vi "Calibration Smoothing Tool.vi"(11 "Path In":path) -> (3 "Smoothed?":bool)   [LabVIEW 2020]
uses:
  Type Defs/Cal-Smoothing Data.ctl
  Type Defs/Cal-Smoothing Parameters.ctl
  SubVIs/Calibration Globals.vi
  Instance           1 28Saved   Calibrate Probe Tube .vi
  PXI DAQ VIs/Utility VIs/Array Dimensions (2D).vi
panel:
  out "save signal":bool=TRUE
  out "Dirty?":bool
  out "plot signal":bool=TRUE
  in  "Tab Control":enum32{"Loess", "MA"}(tab)
  in  "MA":cluster{"Iterations":i32, "Length":i32}={"Iterations"=100, "Length"=3} {"Length" min=1 step=1; "Iterations" min=1 step=1}
  in  "Loess":T1={"Length"=21, "Type"=enum."Quadratic", "Robust"=TRUE} {"Length" min=1 step=1}
  in  "Method":enum16{"Moving average", "Loess"}(ring)=enum."Loess"
  in  "Exit Button":bool
  in  "Apply Button":bool
  in  "Save Button":bool
  in  "Clear Button":bool
  in  "Open Button":bool
  out "exit signal":bool=TRUE
  out "Path":path=path "C:/Data/Probe Tube Calibrations/SN31_ProbeTube.calib"
  out "PT phase graph":cluster{"PTC Mag":dbl[], "PTC Phase":dbl[]}[](graph)
  out "Mag Graph":cluster{"Numeric":dbl, dbl, dbl[][]}(graph)
  # "Smoothing parameters"
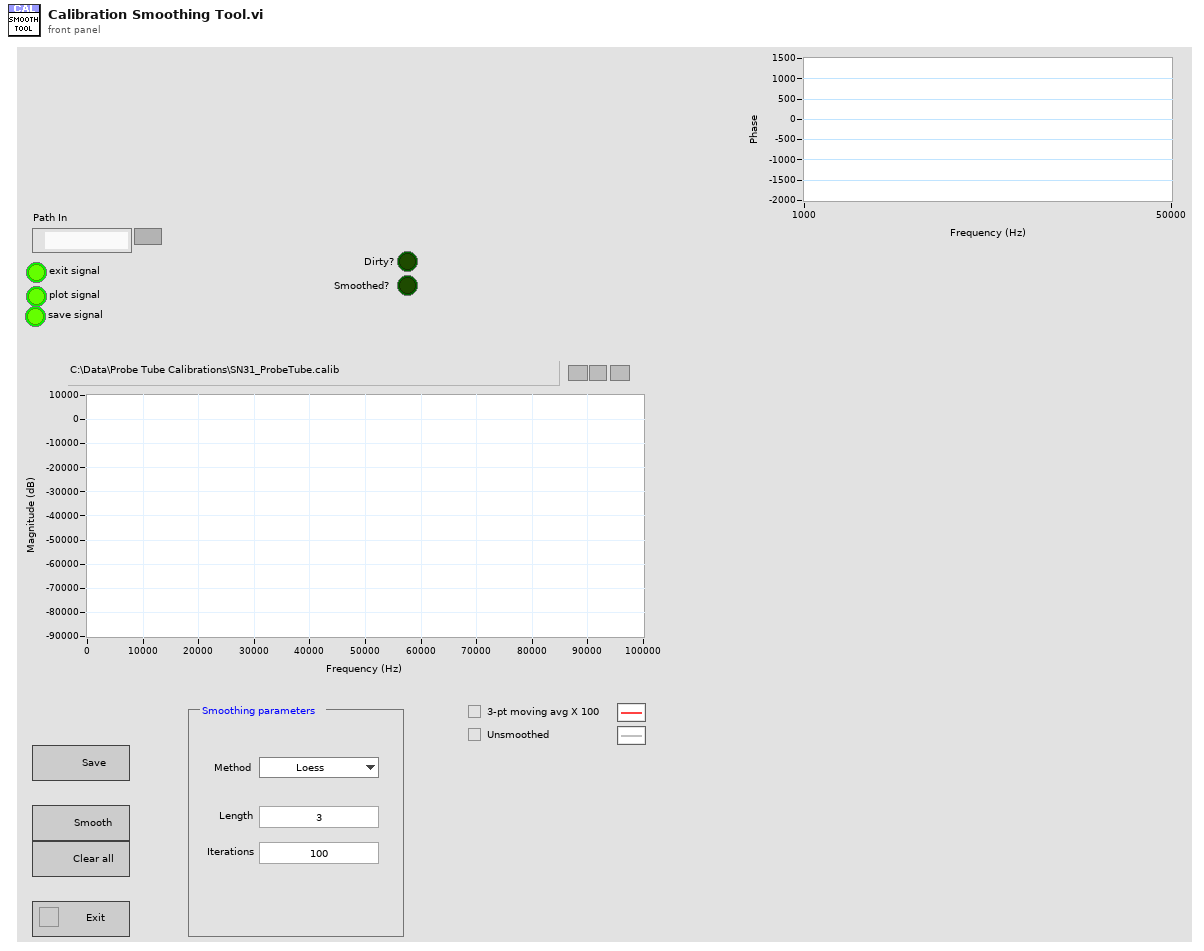
[diagram p1: front panel]
types:
  T1 = cluster{"Length":i32, "Type":enum16{"Linear", "Quadratic"}, "Robust":bool}
  T2 = typedef "Cal-Smoothing Data.ctl" = cluster{"Data":cluster{"x0":dbl, "dx":dbl, "Array":dbl[][]}, "Labels":string[], "Smooth Params":T3}
  T3 = typedef "Cal-Smoothing Parameters.ctl" = cluster{"Method":enum16{"None", "Moving average", "Loess"}, "MA":cluster{"Iterations":i32, "Length":i32}, "Loess":cluster{"Length":i32, "Type":enum16{"Linear", "Quadratic"}, "Robust":bool}}
  T4 = enum16{"Left Button", "Center Button", "Right Button", "Window Close"}
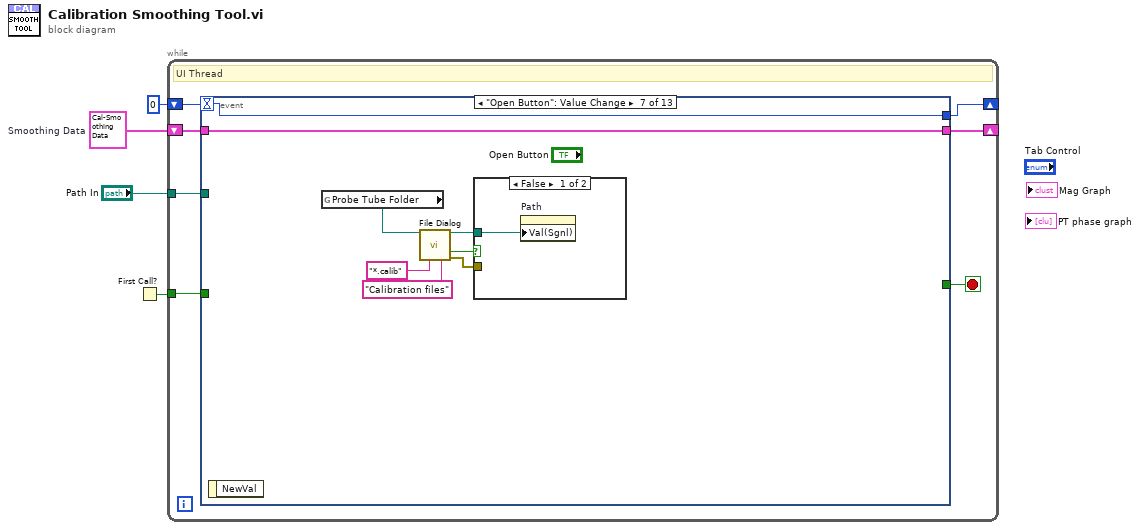
[diagram p0: block diagram]
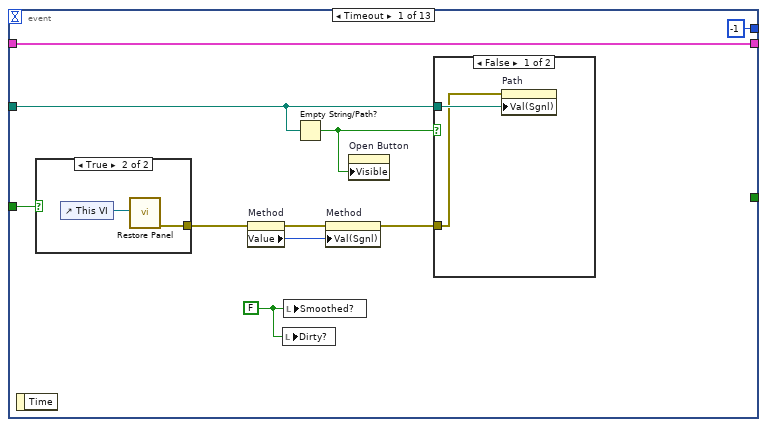
[diagram p2: hidden frame]
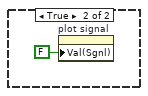
[diagram p3: hidden frame]
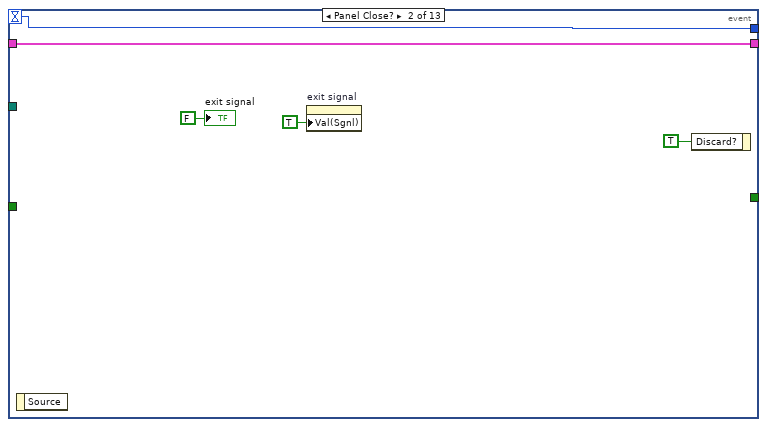
[diagram p5: hidden frame]
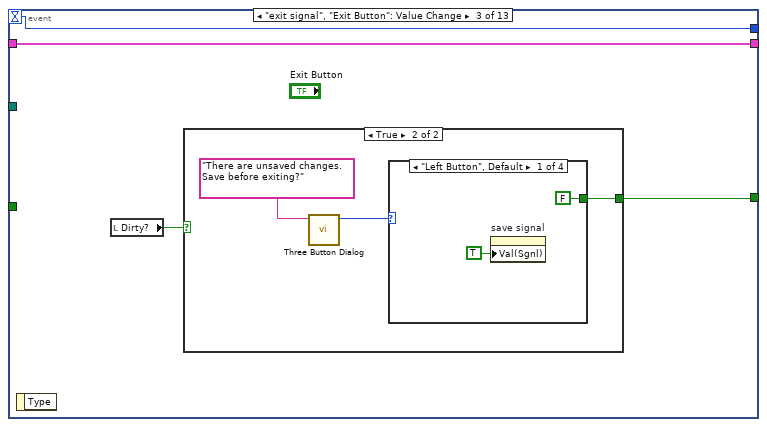
[diagram p6: hidden frame]
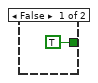
[diagram p7: hidden frame]
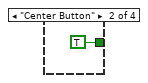
[diagram p8: hidden frame]
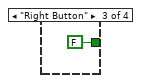
[diagram p9: hidden frame]
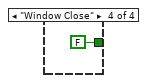
[diagram p10: hidden frame]
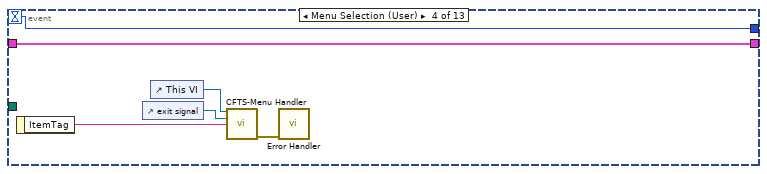
[diagram p11: hidden frame]
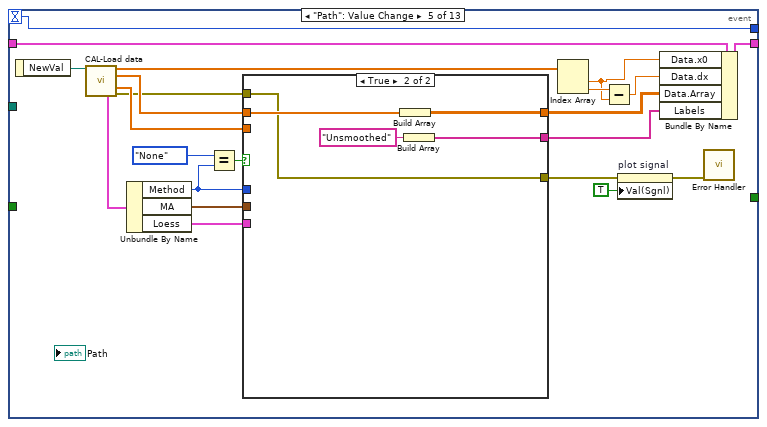
[diagram p12: hidden frame]
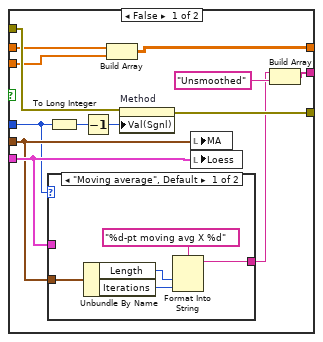
[diagram p13: hidden frame]
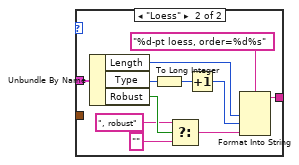
[diagram p14: hidden frame]
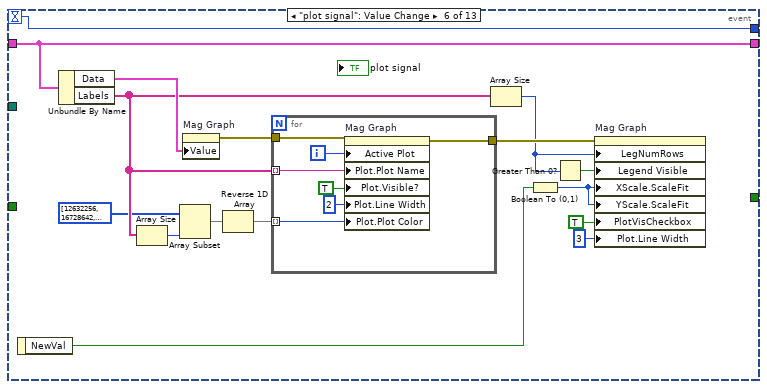
[diagram p15: hidden frame]
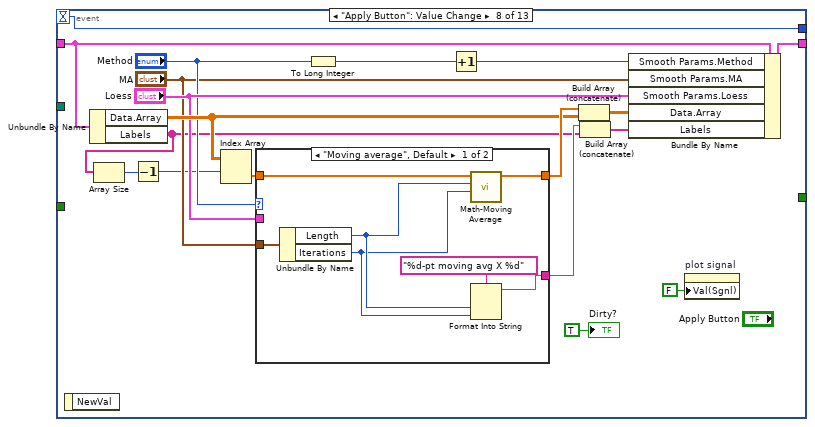
[diagram p17: hidden frame]
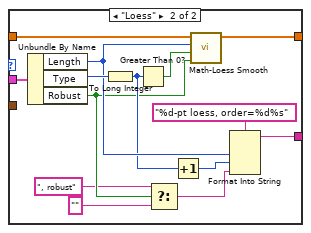
[diagram p18: hidden frame]
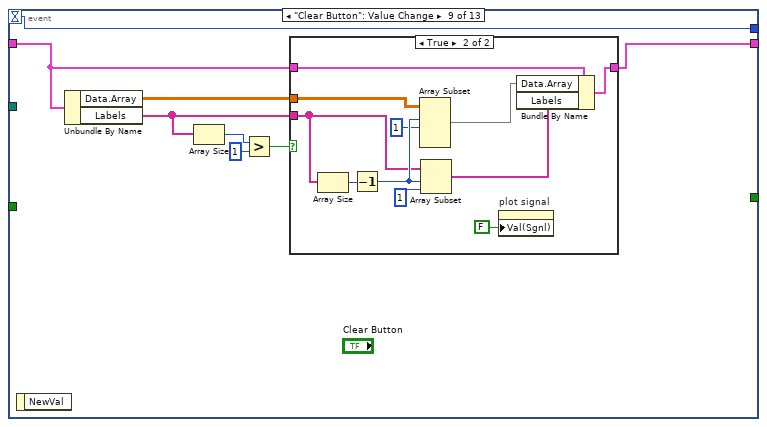
[diagram p19: hidden frame]
diagram:
  w2 = T2 {"Data"={"x0"=0.0, "dx"=0.0, "Array"=[]}, "Labels"=[], "Smooth Params"={"Method"=enum."Loess", "MA"={"Iterations"=100, "Length"=3}, "Loess"={"Length"=21, "Type"=enum."Quadratic", "Robust"=TRUE}}}  # Smoothing Data
  n1 = First Call?() -> (First Call?: T/F=w3:bool)
  n2 = while {
    shift-right: [w9] -> _
    shift-left: 0 -> [w10]
    tunnel: w3 -> [w8]
    shift-right: [w6] -> _
    shift-left: w2 -> [w7]
    tunnel: "Path In" -> [w5]
    stop <- w11 stop-if-true
    # "UI Thread"
    n3 = event shown="[6] \"Open Button\": Value Change" {
      selector: _ -> [_ _ _ _ _ _ _ _ _ _ _ _ _]
      dyn-events: _ -> [_ _ _ _ _ _ _ _ _ _ _ _ _]
      timeout: w10 -> [_ w30 w35 w50 w72 w122 w132 w157 w186 w201 w210 w228 w230]
      tunnel: [_ _ w33 _ _ _ _ _ _ _ w202 _ _] -> w11
      tunnel: [-1 w30 w35 w50 w72 w122 w132 w157 w186 w201 w210 w228 w230] -> w9
      tunnel: w8 -> [w20 _ _ _ _ _ _ _ _ _ _ _ _]
      tunnel: w7 -> [w19 w27 w32 w45 w67 w121 w131 w154 w185 w200 w209 w225 w229]
      tunnel: [w19 w27 w32 w45 w66 w121 w131 w152 w183 w200 w209 w225 w229] -> w6
      tunnel: w5 -> [w15 _ _ _ _ _ _ _ _ _ _ _ _]
      event Timeout {
        w14 = FALSE ("Smoothed?")
        n4 = event-data() -> ()  [unwired: 1 in, 1 out]
        n5 = case shown="True" w20 {
          tunnel: [_ w25] -> w18
          frame False {
          }
          frame True {
            n6 = control-ref of="This VI"() -> (w26:refnum<vi>)
            n7 = call "Restore Panel.vi"("VI reference"=w26) -> ("error out"=w25:errorcluster)  [unwired: 10 in]
          }
        }
        n8 = property on="Method" class="Enum (strict)"(error in=w18) -> (error out=w17:errorcluster, "Value"=w16:enum16{"Moving average", "Loess"})  [unwired: 1 in, 1 out]
        n9 = local write "Dirty?"(w14) -> ()
        n10 = local write "Smoothed?"(w14) -> ()
        n11 = Empty String/Path?(string/path=w15) -> (empty?=w12:bool)
        n12 = property on="Method" class="Enum (strict)"(error in=w17, "Val(Sgnl)"=w16) -> (error out=w13:errorcluster)  [unwired: 1 in, 1 out]
        n13 = property on="Open Button" class="Bool"("Visible"=w12) -> ()  [unwired: 2 in, 2 out]
        n14 = case shown="False" w12 {
          tunnel: w15 -> [w23 _]
          tunnel: w13 -> [w22 _]
          frame False {
            n15 = property on="Path" class="Path"(error in=w22, "Val(Sgnl)"=w23) -> ()  [unwired: 1 in, 2 out]
          }
          frame True {
            n16 = property on="plot signal" class="Bool (strict)"("Val(Sgnl)"=FALSE ("Value (Signaling)")) -> ()  [unwired: 2 in, 2 out]
          }
        }
      }
      event Panel Close? {
        n17 = event-data() -> ()  [unwired: 1 in, 1 out]
        n18 = property on="exit signal" class="Bool (strict)"("Val(Sgnl)"=TRUE ("Value (Signaling)")) -> ()  [unwired: 2 in, 2 out]
        n19 = event-data("Discard?"=TRUE) -> ()  [unwired: 1 in, 1 out]
        "exit signal" <- FALSE ("exit signal")
      }
      event "exit signal", "Exit Button": Value Change {
        n20 = event-data() -> ()  [unwired: 1 in, 1 out]
        n21 = local read "Dirty?"() -> (w34:bool)
        n22 = case shown="True" w34 {
          tunnel: [TRUE w37] -> w33
          frame False {
          }
          frame True {
            n23 = call <vilib>:"Three Button Dialog.vi"("message"="There are unsaved changes. Save before exiting?") -> ("Which Button?"=w38:T4)  [unwired: 10 in]
            n24 = case shown="\"Left Button\", Default" w38 {
              tunnel: [FALSE TRUE FALSE FALSE] -> w37
              frame "Left Button", Default {
                n25 = property on="save signal" class="Bool (strict)"("Val(Sgnl)"=TRUE ("Value (Signaling)")) -> ()  [unwired: 2 in, 2 out]
              }
              frame "Center Button" {
              }
              frame "Right Button" {
              }
              frame "Window Close" {
              }
            }
          }
        }
      }
      event Menu Selection (User) {
        n26 = event-data() -> ("ItemTag"=w47:string)  [unwired: 1 in]
        n27 = control-ref of="exit signal"() -> (w46:refnum<vi>)
        n28 = control-ref of="This VI"() -> (w49:refnum<vi>)
        n29 = call "CFTS-Menu Handler.vi"("VI Refnum"=w49, "Return Refnum"=w46, "ItemTag"=w47) -> ("error out"=w48:errorcluster)  [unwired: 11 in, 1 out]
        n30 = call "Error Handler.vi"("error in (no error)"=w48) -> ()  [unwired: 13 in, 2 out]
      }
      event "Path": Value Change {
        n31 = event-data() -> ("NewVal"=w71:path)  [unwired: 1 in]
        n32 = call "CAL-Load data.vi"("user path"=w71) -> ("Smooth Params"=w59:T3, "Frequency (Hz)"=w69:dbl[], "Mag"=w68:dbl[], "Unsmoothed Mag"=w56:dbl[], "error out"=w52:errorcluster)  [unwired: 7 in, 3 out]
        n33 = Unbundle By Name(w59) -> ("Method"=w53:enum16{"None", "Moving average", "Loess"}, "MA"=w55:cluster{"Iterations":i32, "Length":i32}, "Loess"=w54:T1)
        n34 = Equal?(x=enum16{"None", "Moving average", "Loess"}."None", y=w53) -> (x = y?=w57:bool)
        n35 = case shown="True" w57 {
          tunnel: w68 -> [w84 w106]
          tunnel: [w82 w105] -> w63
          tunnel: [w80 w103] -> w60
          tunnel: w56 -> [w83 _]
          tunnel: w55 -> [w75 _]
          tunnel: w54 -> [w76 _]
          tunnel: w53 -> [w74 _]
          tunnel: w52 -> [w85 w102]
          tunnel: [w77 w102] -> w51
          frame False {
            n36 = case shown="\"Moving average\", Default" w74 {
              tunnel: w76 -> [_ w100]
              tunnel: w75 -> [w90 _]
              tunnel: [w88 w98] -> w73
              frame "Moving average", Default {
                n37 = Unbundle By Name(w90) -> ("Length"=w87:i32, "Iterations"=w86:i32)
                n38 = Format Into String(format string="%d-pt moving avg X %d", w87, w86) -> (resulting string=w88:string)  [unwired: 2 in, 1 out]
              }
              frame "Loess" {
                n39 = Unbundle By Name(w100) -> ("Length"=w97:i32, "Type"=w101:enum16{"Linear", "Quadratic"}, "Robust"=w93:bool)
                n40 = To Long Integer(number=w101) -> (32bit integer=w96:i32)
                n41 = Select(t=", robust", s=w93, f="") -> (s? t:f=w94:string)
                n42 = Increment(x=w96) -> (x+1=w95:i32)
                n43 = Format Into String(format string="%d-pt loess, order=%d%s", w97, w95, w94) -> (resulting string=w98:string)  [unwired: 2 in, 1 out]
              }
            }
            n44 = To Long Integer(number=w74) -> (32bit integer=w79:i32)
            n45 = Decrement(x=w79) -> (x-1=w78:i32)
            n46 = Build Array(w84, w83) -> (w82:dbl[][])
            n47 = property on="Method" class="Enum (strict)"(error in=w85, "Val(Sgnl)"=w78) -> (error out=w77:errorcluster)  [unwired: 1 in, 1 out]
            n48 = local write "MA"(w75) -> ()
            n49 = local write "Loess"(w76) -> ()
            n50 = Build Array(w73, "Unsmoothed") -> (w80:string[])
          }
          frame True {
            n51 = Build Array(w106) -> (w105:dbl[][])
            n52 = Build Array("Unsmoothed" ("String")) -> (w103:string[])
          }
        }
        n53 = Index Array(array=w69) -> (element #1=w65:dbl, element #2=w70:dbl)  [unwired: 2 in]
        n54 = Subtract(x=w70, y=w65) -> (x-y=w64:dbl)
        n55 = property on="plot signal" class="Bool (strict)"(error in=w51, "Val(Sgnl)"=TRUE ("Value (Signaling)")) -> (error out=w62:errorcluster)  [unwired: 1 in, 1 out]
        n56 = Bundle By Name(cluster=w67, "Data.x0"=w65, "Data.dx"=w64, "Data.Array"=w63, "Labels"=w60) -> (w66:T2)
        n57 = call "Error Handler.vi"("error in (no error)"=w62) -> ()  [unwired: 13 in, 2 out]
      }
      event "plot signal": Value Change {
        n58 = event-data() -> ("NewVal"=w119:bool)  [unwired: 1 in]
        n59 = Unbundle By Name(w121) -> ("Data"=w117:cluster{"x0":dbl, "dx":dbl, "Array":dbl[][]}, "Labels"=w111:string[])
        n60 = Array Size(array=w111) -> (size(s)=w110:i32)
        n61 = Array Subset(array=u32[] [12632256, 16728642, 982784, 4375295, 13827953, 13457919, 16757522, 4343295, 16728758, 5898228] ("Array"), length=w110) -> (w108:u32[])  [unwired: 1 in]
        n62 = property on="Mag Graph" class="WFGraph (strict)"("Value"=w117) -> (error out=w118:errorcluster)  [unwired: 2 in, 1 out]
        n63 = Reverse 1D Array(array=w108) -> (reversed array=w107:u32[])
        n64 = for {
          tunnel: w111 -> [w128] mode=indexing
          tunnel: [w127] -> w120
          tunnel: w118 -> [w126]
          tunnel: w107 -> [w123] mode=indexing
          i -> [w129]
          n65 = property on="Mag Graph" class="WFGraph (strict)"(error in=w126, "Active Plot"=w129, "Plot.Plot Name"=w128, "Plot.Visible?"=TRUE ("Plot.Visible"), "Plot.Line Width"=u8 2, "Plot.Plot Color"=w123) -> (error out=w127:errorcluster)  [unwired: 1 in, 1 out]
        }
        n66 = Array Size(array=w111) -> (size(s)=w114:i32)
        n67 = Boolean To (0,1)(Boolean=w119) -> (0, 1=w113:i16)
        n68 = Greater Than 0?(x=w114) -> (x > 0?=w115:bool)
        n69 = property on="Mag Graph" class="WFGraph (strict)"(error in=w120, "LegNumRows"=w114, "Legend Visible"=w115, "XScale.ScaleFit"=w113, "YScale.ScaleFit"=w113, "PlotVisCheckbox"=TRUE ("Legend:Plot Visibility Checkbox Visible"), "Plot.Line Width"=u8 3) -> ()  [unwired: 1 in, 2 out]
      }
      event "Open Button": Value Change {
        n70 = event-data() -> ()  [unwired: 1 in, 1 out]
        n71 = global read "Calibration Globals.vi" "Probe Tube Folder"() -> (w133:path)
        n72 = call "File Dialog"("start path"=w133, "pattern (all files)"="*.calib", "pattern label"="Calibration files") -> ("selected path"=w136:path, "cancelled"=w137:bool, "error out"=w130:errorcluster)  [unwired: 9 in, 1 out]
        n73 = case shown="False" w137 {
          tunnel: w136 -> [w138 _]
          tunnel: w130 -> [_ _]
          frame False {
            n74 = property on="Path" class="Path"("Val(Sgnl)"=w138) -> ()  [unwired: 2 in, 2 out]
          }
          frame True {
          }
        }
      }
      event "Apply Button": Value Change {
        n75 = event-data() -> ()  [unwired: 1 in, 1 out]
        n76 = Unbundle By Name(w154) -> ("Data.Array"=w153:dbl[][], "Labels"=w141:string[])
        n77 = Array Size(array=w141) -> (size(s)=w140:i32)
        n78 = Decrement(x=w140) -> (x-1=w139:i32)
        n79 = Index Array(array=w153, index (row)=w139) -> (element=w156:dbl[])  [unwired: 1 in]
        n80 = case shown="\"Moving average\", Default" "Method" {
          tunnel: w156 -> [w163 w178]
          tunnel: [w162 w177] -> w155
          tunnel: "Loess" -> [_ w174]
          tunnel: "MA" -> [w164 _]
          tunnel: [w160 w172] -> w145
          frame "Moving average", Default {
            n81 = Unbundle By Name(w164) -> ("Length"=w159:i32, "Iterations"=w158:i32)
            n82 = call "Math-Moving Average.vi"("Iterations"=w158, "Length"=w159, "Array in"=w163) -> ("Array out"=w162:dbl[])  [unwired: 8 in]
            n83 = Format Into String(format string="%d-pt moving avg X %d", w159, w158) -> (resulting string=w160:string)  [unwired: 2 in, 1 out]
          }
          frame "Loess" {
            n84 = Unbundle By Name(w174) -> ("Length"=w171:i32, "Type"=w176:enum16{"Linear", "Quadratic"}, "Robust"=w167:bool)
            n85 = To Long Integer(number=w176) -> (32bit integer=w170:i32)
            n86 = Greater Than 0?(x=w170) -> (x > 0?=w175:bool)
            n87 = Select(t=", robust", s=w167, f="") -> (s? t:f=w168:string)
            n88 = Increment(x=w170) -> (x+1=w169:i32)
            n89 = call "Math-Loess Smooth.vi"("Robust?"=w167, "Quadratic?"=w175, "Span"=w171, "Array"=w178) -> ("Smoothed Array"=w177:dbl[])  [unwired: 7 in]
            n90 = Format Into String(format string="%d-pt loess, order=%d%s", w171, w169, w168) -> (resulting string=w172:string)  [unwired: 2 in, 1 out]
          }
        }
        n91 = To Long Integer(number="Method") -> (32bit integer=w144:i32)
        n92 = Increment(x=w144) -> (x+1=w143:i32)
        n93 = Build Array (concatenate)(w155, w153) -> (w149:dbl[][])
        n94 = Build Array (concatenate)(w145, w141) -> (w148:string[])
        n95 = Bundle By Name(cluster=w154, "Smooth Params.Method"=w143, "Smooth Params.MA"="MA", "Smooth Params.Loess"="Loess", "Data.Array"=w149, "Labels"=w148) -> (w152:T2)
        n96 = property on="plot signal" class="Bool (strict)"("Val(Sgnl)"=FALSE ("Value (Signaling)")) -> ()  [unwired: 2 in, 2 out]
        "Dirty?" <- TRUE ("Dirty?")
      }
      event "Clear Button": Value Change {
        n97 = event-data() -> ()  [unwired: 1 in, 1 out]
        n98 = Unbundle By Name(w185) -> ("Data.Array"=w184:dbl[][], "Labels"=w180:string[])
        n99 = Array Size(array=w180) -> (size(s)=w181:i32)
        n100 = Greater?(x=w181, y=1) -> (0:w179:bool)
        n101 = case shown="True" w179 {
          tunnel: w185 -> [w187 w198]
          tunnel: w184 -> [_ w195]
          tunnel: w180 -> [_ w194]
          tunnel: [w187 w191] -> w183
          frame False {
          }
          frame True {
            n102 = Array Size(array=w194) -> (size(s)=w197:i32)
            n103 = Decrement(x=w197) -> (x-1=w196:i32)
            n104 = Array Subset(array=w195, index (row)=w196, length (row)=1 ("length")) -> (w190:dbl[][])  [unwired: 2 in]
            n105 = Array Subset(array=w194, index=w196, length=1) -> (w189:string[])
            n106 = property on="plot signal" class="Bool (strict)"("Val(Sgnl)"=FALSE ("Value (Signaling)")) -> ()  [unwired: 2 in, 2 out]
            n107 = Bundle By Name(cluster=w198, "Data.Array"=w190, "Labels"=w189) -> (w191:T2)
          }
        }
      }
      event "Save Button": Value Change {
        n108 = event-data() -> ()  [unwired: 1 in, 1 out]
        n109 = property on="save signal" class="Bool (strict)"("Val(Sgnl)"=FALSE ("Value (Signaling)")) -> ()  [unwired: 2 in, 2 out]
      }
      event "save signal": Value Change {
        n110 = event-data() -> ("NewVal"=w203:bool)  [unwired: 1 in]
        n111 = Unbundle By Name(w209) -> ("Smooth Params"=w208:T3)
        n112 = Unbundle By Name(w209) -> ("Data.Array"=w207:dbl[][])
        n113 = call-poly "Array Dimensions.vi"("2D Array"=w207) -> ("# rows"=w206:i32)  [unwired: 13 in, 1 out]
        n114 = Greater?(x=w206, y=1) -> (0:w204:bool)
        n115 = case shown="True" w204 {
          tunnel: w208 -> [_ w216]
          tunnel: w207 -> [_ w215]
          tunnel: w203 -> [_ w213]
          tunnel: [FALSE w212] -> w202
          frame False {
          }
          frame True {
            n116 = Index Array(array=w215) -> (element=w217:dbl[])  [unwired: 2 in]
            n117 = local read "Path"() -> (w218:path)
            n118 = call "CAL-Save Smoothed.vi"("path"=w218, "Smoothed"=w217, "Smooth Params"=w216) -> ("error out"=w214:errorcluster)  [unwired: 11 in, 1 out]
            n119 = case shown="No Error" w214 {
              selector: w214 -> [_ w224]
              tunnel: w213 -> [w219 _]
              tunnel: [w219 FALSE ("NewVal")] -> w212
              frame No Error {
                n120 = case shown="False" w219 {
                  frame False {
                    n121 = One Button Dialog(message="Smoothed calibration successfully saved.") -> ()  [unwired: 1 in, 1 out]
                  }
                  frame True {
                  }
                }
                n122 = local write "Dirty?"(FALSE ("Dirty?")) -> ()
                "Smoothed?" <- TRUE ("Smoothed?")
              }
              frame Error {
                n123 = call "Error Handler.vi"("error in (no error)"=w224) -> ()  [unwired: 13 in, 2 out]
              }
            }
          }
        }
      }
      event "Method": Value Change {
        n124 = event-data() -> ("NewVal"=w227:enum16{"Moving average", "Loess"})  [unwired: 1 in]
        n125 = To Long Integer(number=w227) -> (32bit integer=w226:i32)
        n126 = local write "Tab Control"(w226) -> ()
      }
      event "MA.Length": Value Change {
        w235 = 2 ("y")
        n127 = event-data() -> ("NewVal"=w232:i32)  [unwired: 1 in]
        n128 = Divide(x=w232, y=w235) -> (x/y=w237:dbl)
        n129 = Round Toward -Infinity(1:w237) -> (0:w236:dbl)
        n130 = Multiply(x=w236, y=w235) -> (x*y=w234:dbl)
        n131 = To Long Integer(number=w234) -> (32bit integer=w233:i32)
        n132 = Increment(x=w233) -> (x+1=w231:i32)
        n133 = property on="Length" class="DigNum (strict)"("Value"=w231) -> ()  [unwired: 2 in, 2 out]
      }
    }
  }
